vi "dfd_Draw Text.vi"(0 "text orientation":T2(ring), 4 "BG color(transparent)":u32(colorbox)=16777216, 5 "font input":T4={"Font Name:"="", "Size"=12, "Strikeout?"=FALSE, "Italic?"=FALSE, "Underline?"=FALSE, "Outline?"=FALSE, "Shadow?"=FALSE, "Bold?"=FALSE}, 6 "text color(black)":u32(colorbox), 8 "text":string, 9 "alignment(left, top)":T3, 10 "rect in":T1, 11 "picture in":picture) -> (1 "rect out":T1, 3 "picture out":picture)   [LabVIEW 2017, in "NI_DigFilter_Process.lvlib"]
uses:
  <vilib>/addons/Digital Filter Design/NI_DigFilter_Process.lvlib
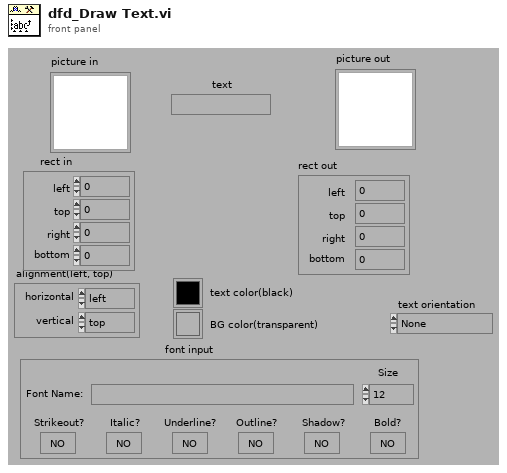
[diagram p1: front panel]
types:
  T1 = cluster{"left":i16, "top":i16, "right":i16, "bottom":i16}
  T2 = enum16{"None", "Stacked", "Clockwise", "Counterclockwise"}
  T3 = cluster{"horizontal":enum16{"left", "center", "right"}, "vertical":enum16{"top", "center", "bottom"}}
  T4 = cluster{"Font Name:":string, "Size":i16, "Strikeout?":bool, "Italic?":bool, "Underline?":bool, "Outline?":bool, "Shadow?":bool, "Bold?":bool}
  T5 = enum16{"User-specified Font", "Application Font", "System Font", "Dialog Font"}
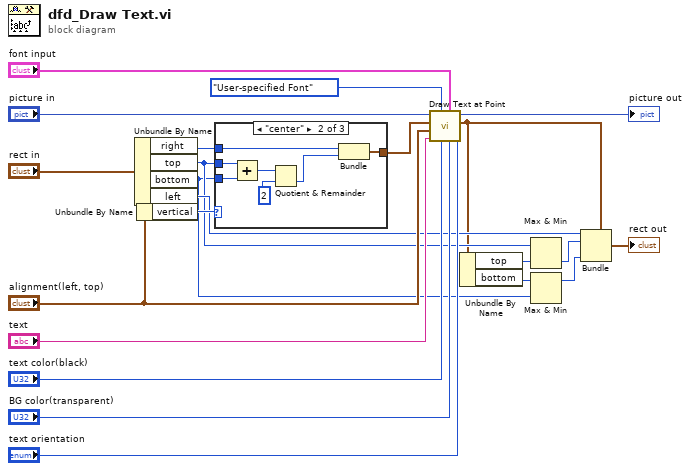
[diagram p0: block diagram]
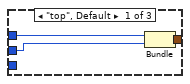
[diagram p2: hidden frame]
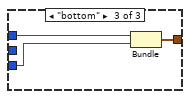
[diagram p3: hidden frame]
diagram:
  n1 = Unbundle By Name("rect in") -> ("right"=w11:i16, "top"=w8:i16, "bottom"=w6:i16, "left"=w9:i16)
  n2 = Unbundle By Name("alignment(left, top)") -> ("vertical"=w12:enum16{"top", "center", "bottom"})
  n3 = case shown="\"center\"" w12 {
    tunnel: w11 -> [w25 w31 w35]
    tunnel: [w24 w32 w33] -> w10
    tunnel: w8 -> [w23 w30 _]
    tunnel: w6 -> [_ w29 w34]
    frame "top", Default {
      n4 = Bundle("right"=w25, "top"=w23) -> (w24:cluster{"right":i16, "top":i16})  [unwired: 1 out]
    }
    frame "center" {
      n5 = Add(x=w30, y=w29) -> (x+y=w28:i16)
      n6 = Quotient & Remainder(x=w28, y=i16 2) -> (floor(x/y)=w26:i16)  [unwired: 1 out]
      n7 = Bundle("right"=w31, w26) -> (w32:cluster{"right":i16, i16})  [unwired: 1 out]
    }
    frame "bottom" {
      n8 = Bundle("right"=w35, "bottom"=w34) -> (w33:cluster{"right":i16, "bottom":i16})  [unwired: 1 out]
    }
  }
  n9 = call <vilib>:"Draw Text at Point.vi"("text orientation"="text orientation", "BG color(transparent)"="BG color(transparent)", "[user-specified font]"="font input", "text color(black)"="text color(black)", "desired font(Application)"=T5."User-specified Font", "text"="text", "alignment(left, top)"="alignment(left, top)", "origin"=w10, "picture"="picture in") -> ("text rect"=w4:T1, "new picture"=→"picture out":picture)  [unwired: 1 out]
  n10 = Unbundle By Name(w4) -> ("top"=w7:i16, "bottom"=w5:i16)
  n11 = Max & Min(x=w8, y=w7) -> (min(x,y)=w3:i16)  [unwired: 1 out]
  n12 = Max & Min(x=w5, y=w6) -> (max(x,y)=w2:i16)  [unwired: 1 out]
  n13 = Bundle(cluster=w4, "left"=w9, "top"=w3, "bottom"=w2) -> (→"rect out":T1)  [unwired: 1 out]
